vi "Template - Counter Acquire Frequency.vi"() -> ()   [LabVIEW 2013]
doc: "This example shows how to acquire frequency using the VIs of the driver."
uses:
  <instrlib>/_Template - Counter/Public/Configure/Configure Measurement (Frequency).vi
  <instrlib>/_Template - Counter/Template - Counter.lvlib
panel:
  in  "Timeout (10000 ms)":u32=10000
  out "Frequency":dbl
  in  "VISA resource name":refnum<visa-resource-name>
  # "(c) 2009 <Enter Company Name Here>.  ALL RIGHTS RESERVED."
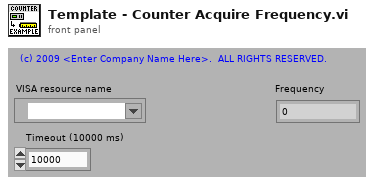
[diagram p1: front panel]
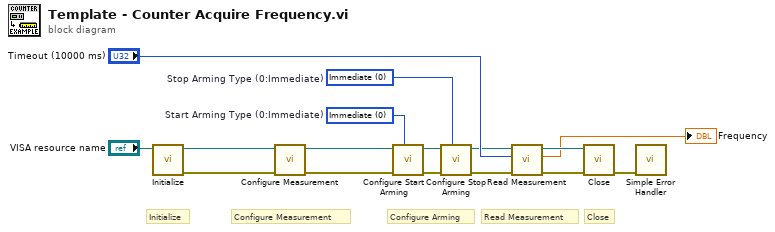
[diagram p0: block diagram]
diagram:
  w7 = 0 items=["Immediate", "External"]  # Start Arming Type (0:Immediate)
  w8 = 0 items=["Immediate", "External"]  # Stop Arming Type (0:Immediate)
  # "Close"
  # "Read Measurement"
  # "Initialize"
  # "Configure Measurement"
  # "Configure Arming"
  n1 = call <instrlib>:"Initialize.vi"("VISA resource name"="VISA resource name") -> ("error out"=w1:errorcluster, "VISA resource name out"=w2:refnum<visa-resource-name>)  [unwired: 9 in]
  n2 = call-poly <instrlib>:"Configure Measurement.vi"("error in (no error)"=w1, "VISA resource name"=w2) -> ("error out"=w3:errorcluster, "VISA resource name out"=w4:refnum<visa-resource-name>)  [unwired: 8 in]
  n3 = call <instrlib>:"Configure Start Arming.vi"("Start Arming Type (0:Immediate)"=w7, "error in (no error)"=w3, "VISA resource name"=w4) -> ("error out"=w13:errorcluster, "VISA resource name out"=w16:refnum<visa-resource-name>)  [unwired: 7 in]
  n4 = call <instrlib>:"Configure Stop Arming.vi"("Stop Arming Type (0:Immediate)"=w8, "error in (no error)"=w13, "VISA resource name"=w16) -> ("error out"=w5:errorcluster, "VISA resource name out"=w6:refnum<visa-resource-name>)  [unwired: 7 in]
  n5 = call <instrlib>:"Read Measurement.vi"("error in (no error)"=w5, "Timeout (10000 ms)"="Timeout (10000 ms)", "VISA resource name"=w6) -> ("error out"=w14:errorcluster, "Measurement"=→"Frequency":dbl, "VISA resource name out"=w15:refnum<visa-resource-name>)  [unwired: 6 in]
  n6 = call <instrlib>:"Close.vi"("error in (no error)"=w14, "VISA resource name"=w15) -> ("error out"=w11:errorcluster)  [unwired: 9 in]
  n7 = call <vilib>:"Simple Error Handler.vi"("error in (no error)"=w11) -> ()  [unwired: 4 in, 5 out]
